vi "error handler.vi"(8 "error in (no error)":errorcluster, 11 "Boolean in":refnum<vi>) -> (0 "error out":errorcluster)   [LabVIEW 2017]
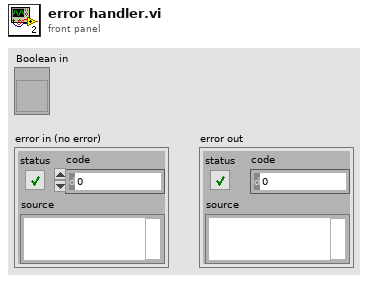
[diagram p1: front panel]
types:
  T1 = enum8{"Enabled", "Disabled", "Disabled and Grayed Out"}
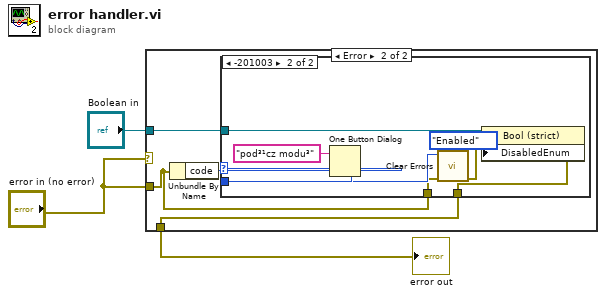
[diagram p0: block diagram]
diagram:
  n1 = case shown="Error" "error in (no error)" {
    tunnel: "error in (no error)" -> [w4 w7]
    tunnel: [w4 w6] -> w3
    tunnel: "Boolean in" -> [_ w5]
    frame No Error {
    }
    frame Error {
      n2 = Unbundle By Name(w7) -> ("code"=w8:i32)
      n3 = case shown="-201003" w8 {
        tunnel: w8 -> [_ w16]
        tunnel: w7 -> [w9 w15]
        tunnel: [w9 w12] -> w6
        tunnel: w5 -> [_ w10]
        frame 0, Default {
        }
        frame -201003 {
          n4 = One Button Dialog(message="pod³¹cz modu³") -> ()  [unwired: 1 in, 1 out]
          n5 = call <vilib>:"Clear Errors.vi"("error in (no error)"=w15, "specific error code to clear (0: all)"=w16) -> ("error out"=w13:errorcluster)  [unwired: 4 in, 1 out]
          n6 = property on="Property Node" class="Bool (strict)"(reference=w10, error in=w13, "DisabledEnum"=T1."Enabled" ("Disabled")) -> (error out=w12:errorcluster)  [unwired: 1 out]
        }
      }
    }
  }
  "error out" <- w3
